vi "medicion_remota_lectura_02.vi"() -> ()   [LabVIEW 2020]
uses:
  <vilib>/httpClient/LabVIEWHTTPClient.lvlib
panel:
  out "Temperatura":dbl
  out "error out 2":errorcluster
  out "Frontal":bool
  out "Lateral":bool
  out "Humedad":dbl
  out "headers":string
  out "body":string
  out "error out":errorcluster
  out "Fecha":string
  in  "stop":bool
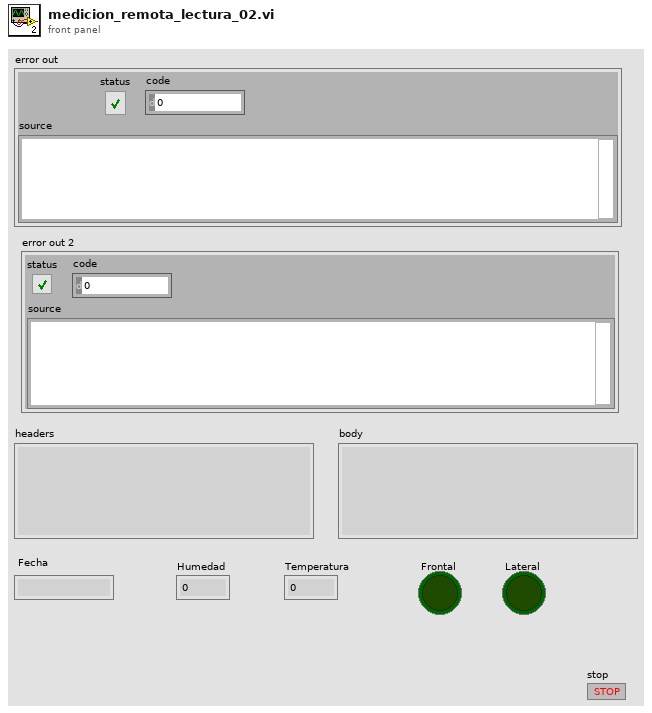
[diagram p1: front panel]
types:
  T1 = cluster{"Humedad":dbl, "Fecha":string, "Temperatura":dbl}
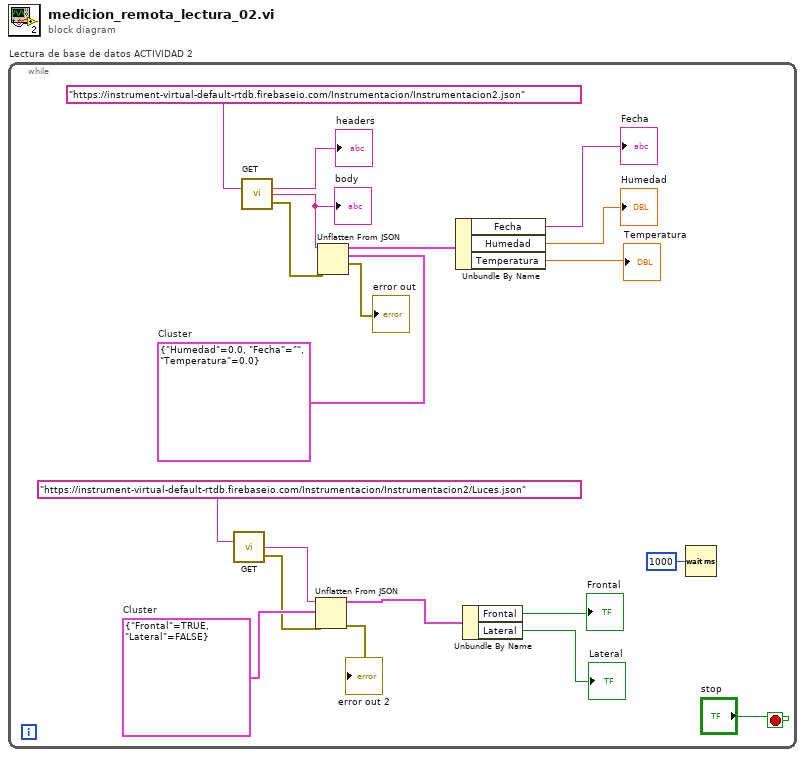
[diagram p0: block diagram]
diagram:
  n1 = while "Lectura de base de datos ACTIVIDAD 2" {
    stop <- "stop" stop-if-true
    w7 = cluster{"Frontal":bool, "Lateral":bool} {"Frontal"=TRUE, "Lateral"=FALSE}  # Cluster
    w16 = T1 {"Humedad"=0.0, "Fecha"="", "Temperatura"=0.0}  # Cluster
    n2 = call <vilib>:"GET.vi"("url"="https://instrument-virtual-default-rtdb.firebaseio.com/Instrumentacion/Instrumentacion2/Luces.json") -> ("body"=w6:string, "error out"=w5:errorcluster)  [unwired: 11 in, 2 out]
    n3 = call <vilib>:"GET.vi"("url"="https://instrument-virtual-default-rtdb.firebaseio.com/Instrumentacion/Instrumentacion2.json") -> ("headers"=→"headers":string, "body"=w15:string, "error out"=w14:errorcluster)  [unwired: 11 in, 1 out]
    "body" <- w15
    n4 = Unflatten From JSON(JSON string=w6, type and defaults=w7, error in (no error)=w5) -> (value=w4:cluster{"Frontal":bool, "Lateral":bool}, error out=→"error out 2":errorcluster)  [unwired: 4 in]
    n5 = Unflatten From JSON(JSON string=w15, type and defaults=w16, error in (no error)=w14) -> (value=w13:T1, error out=→"error out":errorcluster)  [unwired: 4 in]
    n6 = Unbundle By Name "Unbundle By Name"(w13) -> ("Fecha"=→"Fecha":string, "Humedad"=→"Humedad":dbl, "Temperatura"=→"Temperatura":dbl)
    n7 = Unbundle By Name "Unbundle By Name"(w4) -> ("Frontal"=→"Frontal":bool, "Lateral"=→"Lateral":bool)
    n8 = Wait (ms)(milliseconds to wait=u32 1000) -> ()  [unwired: 1 out]
  }
